vi "DHE_GBLDriverVariables.vi"() -> ()   [LabVIEW 2016]
uses:
  DBSHAND/private/vis/DatabaseHand_RefNum.ctl
  Common/public/vis/CMN_TimingInfo.ctl
panel:
  in  "DHE_Nbufs":u16
  out "DHE_ModRef":refnum<vi>
  out "DHE_buff_error":errorcluster
  in  "DHE_post_expose_frames":u16=1
  in  "DHE_pre_expose_frames":u16
  in  "DHE_bpp":i32=131072
  in  "DHE_raw_buffer_size":i32=131072
  in  "DHE_ActiveDevice":string
  in  "DHE_ConfigFile":path
  in  "DHE_TimingInfo":T1={"PixelTime"=1.0, "SkipPixel"=1.0, "SkipRow"=1.0, "ShiftRow"=1.0, "ShiftedPix"=1, "known_overhead"=1.0, "DET_READ_TIME"=1.0} {"DET_READ_TIME" format="%.2f"; "known_overhead" format="%.2f"; "ShiftRow" format="%.2f"; "SkipRow" format="%.2f"; "SkipPixel" format="%.2f"; "PixelTime" format="%.2f"}
  in  "DHE_Status":string="NOT INITIALIZED"
  in  "DHE_InitMacro":path
  in  "DHE_MacroDir":path
  in  "DHE_DetYSize":i32
  in  "DHE_DetXSize":i32
  in  "DHE_log":bool
  out "DHE_DBSRef":T2
  in  "DHE_Algors_file":path=path "/home/arcconfig/ALGORS.list"
  in  "DHE_TP.cfg":path=path "/home/acconfig/TP_DHE.list"
  in  "DHE_bpp":i32=16
  in  "DHE_modifiers":string
  in  "DHE_readmode":string
  in  "DHE_FPA_name":string
  in  "DHE_CommandsToExecute":string[](array[string])
  out "DHE_readout_ended":bool
  in  "DHE_LogFile":path
  in  "DHE_Image Error":T3
  in  "DHE_ModuleName":string
  in  "DHE_ControllerConfigCluster":T4
  in  "DHE_ImgState":T5(ring)
  # "(mS)"
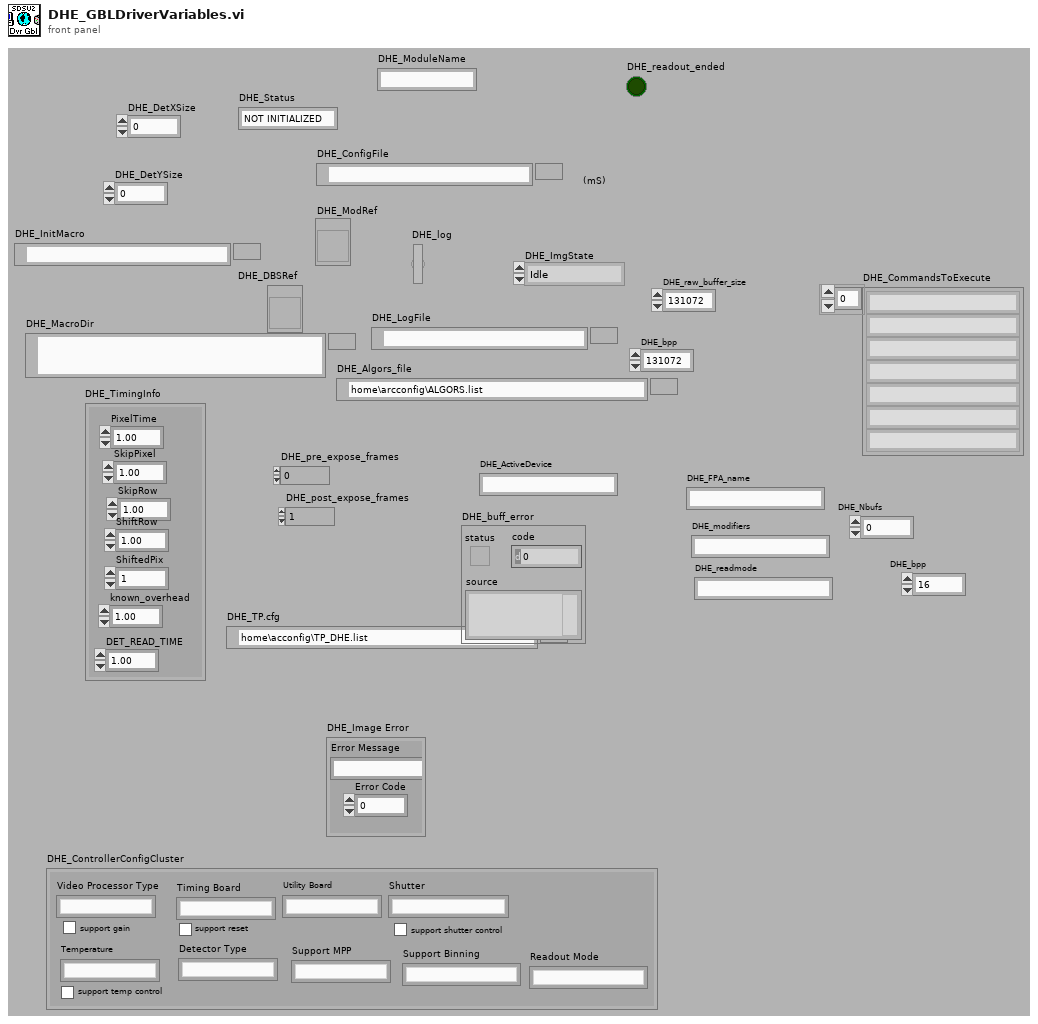
[diagram p1: front panel]
types:
  T1 = typedef "CMN_TimingInfo.ctl" = cluster{"PixelTime":sgl, "SkipPixel":sgl, "SkipRow":sgl, "ShiftRow":sgl, "ShiftedPix":u16, "known_overhead":sgl, "DET_READ_TIME":sgl}
  T2 = typedef "DatabaseHand_RefNum.ctl" = refnum<vi>
  T3 = cluster{"Error Message":string, "Error Code":i32}
  T4 = cluster{"Video Processor Type":string, "support gain":bool, "Timing Board":string, "support reset":bool, "Utility Board":string, "Shutter":string, "Temperature":string, "support temp control":bool, "Detector Type":string, "Support MPP":string, "Support Binning":string, "Readout Mode":string, "support shutter control":bool}
  T5 = enum16{"Idle", "Exposing", "Paused", "AbortExp", "Reading", "AbortRead", "FinishedReading", "Resetting", "Reducing", "Initializing"}
diagram:
